vi "xiCam - GetParam_String.vi"(7 "PRM":T1, 8 "error in (no error)":errorcluster, 11 "xiCam In":refnum<k24>) -> (0 "error out":errorcluster, 3 "xiCam Out":refnum<k24>, 4 "String_Value":string)   [LabVIEW 2016]
doc: "This function returns parameters information (current value, minimum, maximum, info).\n\n<b>String GetParamString(string prm)</b>\nstring prm : Parameter name string. Use class PRM to set parameters.\nReturn : String value to be returned."
uses:
  C:/Users/Ries Lab/Documents/Microscope Control from Sheng Account/Microscope-Control/Device Library/Cameras/Ximea/xiLIB_64bit/xiLIB/xiCamLib/API/x64/xiApi.NETX64.dll
  API/x64/xiApi.NETX64.dll
  PRM/PRM/PRM_v2.ctl
  PRM/BUFF_POLICY/BUFF_POLICY.ctl
  PRM/DOWNSAMPLING_TYPE/DOWNSAMPLING_TYPE.ctl
  PRM/GPI_MODE/GPI_MODE.ctl
  PRM/GPO_MODE/GPO_MODE.ctl
  PRM/IMG_FORMAT/IMG_DATA_FORMAT.ctl
  PRM/LED_MODE/LED_MODE.ctl
  PRM/TRG_SOURCE/TRG_SOURCE.ctl
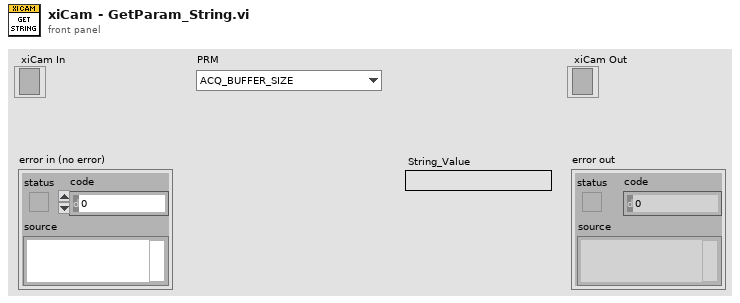
[diagram p1: front panel]
types:
  T1 = typedef "PRM_v2.ctl" = enum16{"ACQ_BUFFER_SIZE", "ACQ_FRAME_BURST_COUNT", "ACQ_TIMING_MODE", "ACQ_TRANSPORT_BUFFER_SIZE", "AE_MAX_LIMIT", "AEAG", "AEAG_LEVEL", "API_VERSION", "AG_MAX_LIMIT", "APPLY_CMS", "AUTO_BANDWIDTH_CALCULATION", "AUTO_WB", "AVAILABLE_BANDWIDTH", "AVAILABLE_BANDWIDTH_MAX", "AVAILABLE_BANDWIDTH_MIN", "BUFFER_POLICY", "BUFFERS_QUEUE_SIZE", "CC_MATRIX_00", "CC_MATRIX_01", "CC_MATRIX_02", "CC_MATRIX_03", "CC_MATRIX_10", "CC_MATRIX_11", "CC_MATRIX_12", "CC_MATRIX_13", "CC_MATRIX_20", "CC_MATRIX_21", "CC_MATRIX_22", "CC_MATRIX_23", "CC_MATRIX_30", "CC_MATRIX_31", "CC_MATRIX_32", "CC_MATRIX_33", "CHIP_TEMP", "CMS", "COLOR_FILTER_ARRAY", "COOLING", "DEBOUNCE_EN", "DEBOUNCE_POL", "DEBOUNCE_T0", "DEBOUNCE_T1", "DEBUG_LEVEL", "DEFAULT_CC_MATRIX", "DEVICE_INSTANCE_PATH", "DEVICE_MODEL_ID", "DEVICE_NAME", "DEVICE_SN", "DEVICE_TYPE", "DEVICE_USER_ID", "DOWNSAMPLING", "DOWNSAMPLING_TYPE", "DRV_VERSION", "EXP_PRIORITY", "EXPOSURE", "EXPOSURE_MAX", "EXPOSURE_MIN", "FFS_FILE_NAME", "FPGA1_VERSION", "FRAMERATE", "FRAMERATE_MAX", "FRAMERATE_MIN", "FREE_FFS_SIZE", "GAIN", "GAIN_MAX", "GAIN_MIN", "GAMMAC", "GAMMAY", "GPI_LEVEL", "GPI_MODE", "GPI_SELECTOR", "GPO_MODE", "GPO_SELECTOR", "HDR", "HDR_T1", "HDR_T2", "HEIGHT", "HEIGHT_MAX", "HEIGHT_MIN", "HOUSE_TEMP", "IMAGE_DATA_FORMAT", "IMAGE_IS_COLOR", "INPUT_CMS_PROFILE", "IS_COOLED", "IS_DEVICE_EXIST", "KNEEPOINT1", "KNEEPOINT2", "LED_MODE", "LED_SELECTOR", "LIMIT_BANDWIDTH", "LIMIT_BANDWIDTH_MAX", "LIMIT_BANDWIDTH_MIN", "LUT_EN", "LUT_INDEX", "LUT_INDEX_MAX", "LUT_INDEX_MIN", "LUT_VALUE", "LUT_VALUE_MAX", "LUT_VALUE_MIN", "MANUAL_WB", "MCU1_VERSION", "MCU2_VERSION", "OFFSET_X", "OFFSET_X_MAX", "OFFSET_X_MIN", "OFFSET_Y", "OFFSET_Y_MAX", "OFFSET_Y_MIN", "OUTPUT_CMS_PROFILE", "OUTPUT_DATA_BIT_DEPTH", "OUTPUT_DATA_PACKING", "READ_FILE_FFS", "RECENT_FRAME", "SENSOR_DATA_BIT_DEPTH", "SENSOR_MODE", "SENSOR_TAPS", "SHARPNESS", "SHUTTER_TYPE", "TARGET_TEMP", "TRG_DELAY", "TRG_SELECTOR", "TRG_SOFTWARE", "TRG_SOURCE", "USED_FFS_SIZE", "WB_KB", "WB_KG", "WB_KR", "WIDTH", "WIDTH_MAX", "WIDTH_MIN", "WRITE_FILE_FFS", "ACQ_BUFFER_SIZE_UNIT", "ACQ_TRANSPORT_BUFFER_COMMIT", "AEAG_ROI_HEIGHT", "AEAG_ROI_OFFSET_X", "AEAG_ROU_OFFSET_Y", "AEAG_ROI_WIDTH", "API_CONTEXT_LIST", "BINNING_HORIZONTAL", "BINNING_SELECTOR", "BINNING_VERTICAL", "COLUMN_FPN_CORRECTION", "COUNTER_SELECTOR", "COUNTER_VALUE", "DECIMATION_HORIZONTAL", "DECIMATION_SELECTOR", "DECIMATION_VERTICAL", "DEVICE_ID", "DEVICE_LOCATION_PATH", "DEVICE_MANIFEST", "DEVICE_RESET", "DEVICE_SENS_SN", "EXPOSURE_BURST_COUNT", "FFS_ACCESS_KEY", "GAIN_SELECTOR", "HW_REVISION", "IMAGE_BLACK_LEVEL", "IMAGE_DATA_BIT_DEPTH", "IMAGE_DATA_FORMAT_RGB32_ALPHA", "IMAGE_PAYLOAD_SIZE", "LENS_APERTURE_VALUE", "LENS_FEATURE", "LENS_FEATURE_SELECTOR", "LENS_FOCAL_LENGTH", "LENS_FOCUS_DISTANCE", "LENS_FOCUS_MOVE", "LENS_FOCUS_MOVEMENT_VALUE", "LENS_MODE", "OUTPUT_DATA_PACKING_TYPE", "SENSOR_CLOCK_FREQ_HZ", "SENSOR_CLOCK_FREQ_INDEX", "SENSOR_FEATURE_SELECTOR", "SENSOR_FEATURE_VALUE", "SENSOR_OUTPUT_CHANNEL_COUNT", "TRANSPORT_PIXEL_FORMAT", "TS_RST_MODE", "TS_RST_SOURCE", "SENS_DEFECTS_CORR_LIST_SELECTOR", "SENS_DEFECTS_CORR", "SENS_DEFECTS_CORR_LIST_CONTENT", "DEVICE_UNIT_SELECTOR", "DEVICE_UNIT_REGISTER_SELECTOR", "DEVICE_UNIT_REGISTER_VALUE"}
  T2 = typedef "BUFF_POLICY.ctl" = enum16{"UNSAFE", "SAFE"}
  T3 = typedef "DOWNSAMPLING_TYPE.ctl" = enum16{"BINNING", "SKIPPING"}
  T4 = typedef "GPI_MODE.ctl" = enum16{"OFF", "TRIGGER", "EXT_EVENT"}
  T5 = typedef "GPO_MODE.ctl" = enum16{"OFF", "ON", "FRAME_ACTIVE", "FRAME_ACTIVE_NEG", "EXPOSURE_ACTIVE", "EXPOSURE_ACTIVE_NEG"}
  T6 = typedef "IMG_DATA_FORMAT.ctl" = enum16{"MONO8", "MONO16", "RGB24", "RGB32", "RGBPLANAR", "RAW8", "RAW16"}
  T7 = typedef "LED_MODE.ctl" = enum16{"HEARTBEAT", "TRIGGER_ACTIVE", "EXT_EVENT_ACTIVE", "ACQUSITION", "EXPOSURE_ACTIVE", "FRAME_ACTIVE", "LINK", "OFF", "ON"}
  T8 = typedef "TRG_SOURCE.ctl" = enum16{"OFF", "EDGE_RISING", "EDGE_FALLING", "SOFTWARE"}
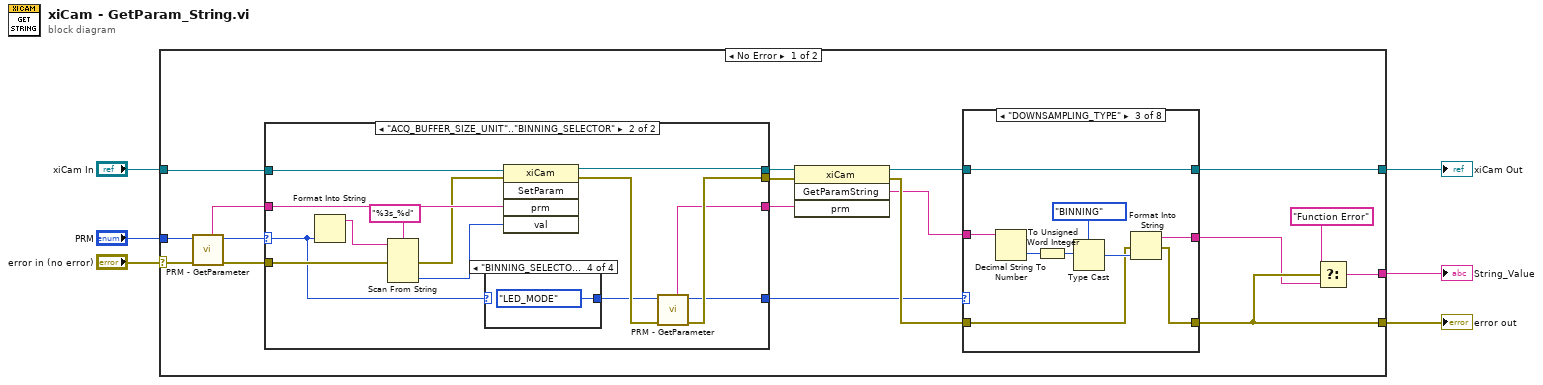
[diagram p0: block diagram]
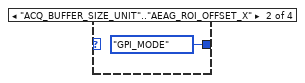
[diagram p4: hidden frame]
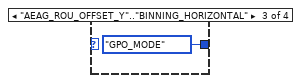
[diagram p5: hidden frame]
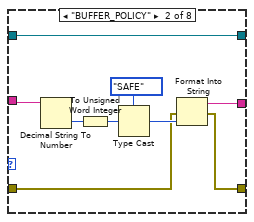
[diagram p7: hidden frame]
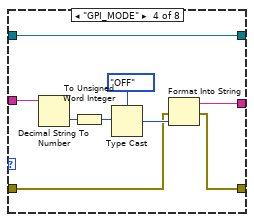
[diagram p8: hidden frame]
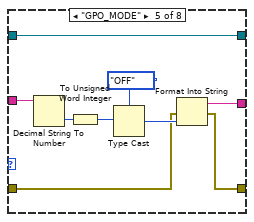
[diagram p9: hidden frame]
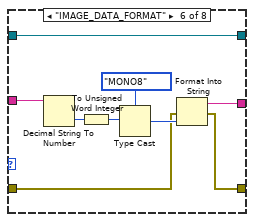
[diagram p10: hidden frame]
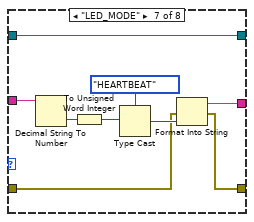
[diagram p11: hidden frame]
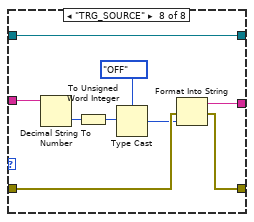
[diagram p12: hidden frame]
diagram:
  n1 = case shown="No Error" "error in (no error)" {
    selector: "error in (no error)" -> [w15 w112]
    tunnel: "xiCam In" -> [w17 w113]
    tunnel: [w21 w113] -> w4
    tunnel: [w10 w112] -> w3
    tunnel: "PRM" -> [w16 _]
    tunnel: [w8 _] -> w1
    frame No Error {
      n2 = call "PRM - GetParameter.vi"("error in (no error)"=w15, "PRM"=w16) -> ("error out"=w19:errorcluster, "PRM OUT"=w18:T1, "ParameterString"=w20:string)  [unwired: 7 in]
      n3 = case shown="\"ACQ_BUFFER_SIZE_UNIT\"..\"BINNING_SELECTOR\"" w18 {
        selector: w18 -> [w25 w34]
        tunnel: w20 -> [w26 w42]
        tunnel: w17 -> [w28 w41]
        tunnel: w19 -> [w27 w38]
        tunnel: [w28 w40] -> w14
        tunnel: [w27 w31] -> w13
        tunnel: [w26 w30] -> w12
        tunnel: [w25 w29] -> w11
        frame Default {
        }
        frame "ACQ_BUFFER_SIZE_UNIT".."BINNING_SELECTOR" {
          n4 = Format Into String(w34) -> (resulting string=w37:string)  [unwired: 3 in, 1 out]
          n5 = Scan From String(format string="%3s_%d", input string=w37, error in=w38) -> (error out=w35:errorcluster, output 2=w36:i32)  [unwired: 4 in, 2 out]
          n6 = case shown="\"BINNING_SELECTOR\"..\"DEVICE_RESET\"" w34 {
            tunnel: [_ PRM_v2."GPI_MODE" ("PRM") PRM_v2."GPO_MODE" ("PRM") PRM_v2."LED_MODE" ("PRM")] -> w32
            frame Default {
            }
            frame "ACQ_BUFFER_SIZE_UNIT".."AEAG_ROI_OFFSET_X" {
            }
            frame "AEAG_ROU_OFFSET_Y".."BINNING_HORIZONTAL" {
            }
            frame "BINNING_SELECTOR".."DEVICE_RESET" {
            }
          }
          n7 = invoke class="xiCam" method="SetParam"(reference=w41, error in=w35, "prm"=w42, "val"=w36) -> (reference out=w40:refnum<k24>, error out=w33:errorcluster)  [unwired: 1 in, 3 out]
          n8 = call "PRM - GetParameter.vi"("error in (no error)"=w33, "PRM"=w32) -> ("error out"=w31:errorcluster, "PRM OUT"=w29:T1, "ParameterString"=w30:string)  [unwired: 7 in]
        }
      }
      n9 = invoke class="xiCam" method="GetParamString"(reference=w14, error in=w13, "prm"=w12) -> (reference out=w23:refnum<k24>, error out=w24:errorcluster, "GetParamString"=w22:string)  [unwired: 1 in, 1 out]
      n10 = case shown="\"DOWNSAMPLING_TYPE\"" w11 {
        tunnel: w24 -> [w47 w54 w64 w73 w82 w91 w100 w110]
        tunnel: w23 -> [w48 w56 w66 w75 w84 w93 w102 w111]
        tunnel: w22 -> [w46 w51 w60 w69 w78 w87 w96 w107]
        tunnel: [w48 w56 w66 w75 w84 w93 w102 w111] -> w21
        tunnel: [w47 w53 w63 w72 w81 w90 w99 w109] -> w10
        tunnel: [w46 w52 w62 w71 w80 w89 w98 w108] -> w9
        frame Default {
        }
        frame "BUFFER_POLICY" {
          n11 = Decimal String To Number(string=w51) -> (number=w50:i32)  [unwired: 2 in, 1 out]
          n12 = To Unsigned Word Integer(number=w50) -> (unsigned 16bit integer=w49:u16)
          n13 = Type Cast(type=BUFF_POLICY."SAFE" ("BUFF_POLICY"), x=w49) -> (*(type *) &x=w55:T2)
          n14 = Format Into String(error in=w54, w55) -> (resulting string=w52:string, error out=w53:errorcluster)  [unwired: 2 in]
        }
        frame "DOWNSAMPLING_TYPE" {
          n15 = Decimal String To Number(string=w60) -> (number=w59:i32)  [unwired: 2 in, 1 out]
          n16 = To Unsigned Word Integer(number=w59) -> (unsigned 16bit integer=w58:u16)
          n17 = Type Cast(type=DOWNSAMPLING_TYPE."BINNING" ("Downsampling Type"), x=w58) -> (*(type *) &x=w65:T3)
          n18 = Format Into String(error in=w64, w65) -> (resulting string=w62:string, error out=w63:errorcluster)  [unwired: 2 in]
        }
        frame "GPI_MODE" {
          n19 = Decimal String To Number(string=w69) -> (number=w68:i32)  [unwired: 2 in, 1 out]
          n20 = To Unsigned Word Integer(number=w68) -> (unsigned 16bit integer=w67:u16)
          n21 = Type Cast(type=GPI_MODE."OFF" ("GPI_MODE"), x=w67) -> (*(type *) &x=w74:T4)
          n22 = Format Into String(error in=w73, w74) -> (resulting string=w71:string, error out=w72:errorcluster)  [unwired: 2 in]
        }
        frame "GPO_MODE" {
          n23 = Decimal String To Number(string=w78) -> (number=w77:i32)  [unwired: 2 in, 1 out]
          n24 = To Unsigned Word Integer(number=w77) -> (unsigned 16bit integer=w76:u16)
          n25 = Type Cast(type=GPO_MODE."OFF" ("GPO_MODE"), x=w76) -> (*(type *) &x=w83:T5)
          n26 = Format Into String(error in=w82, w83) -> (resulting string=w80:string, error out=w81:errorcluster)  [unwired: 2 in]
        }
        frame "IMAGE_DATA_FORMAT" {
          n27 = Decimal String To Number(string=w87) -> (number=w86:i32)  [unwired: 2 in, 1 out]
          n28 = To Unsigned Word Integer(number=w86) -> (unsigned 16bit integer=w85:u16)
          n29 = Type Cast(type=IMG_DATA_FORMAT."MONO8" ("IMG_FORMAT"), x=w85) -> (*(type *) &x=w92:T6)
          n30 = Format Into String(error in=w91, w92) -> (resulting string=w89:string, error out=w90:errorcluster)  [unwired: 2 in]
        }
        frame "LED_MODE" {
          n31 = Decimal String To Number(string=w96) -> (number=w95:i32)  [unwired: 2 in, 1 out]
          n32 = To Unsigned Word Integer(number=w95) -> (unsigned 16bit integer=w94:u16)
          n33 = Type Cast(type=LED_MODE."HEARTBEAT" ("LED_MODE"), x=w94) -> (*(type *) &x=w101:T7)
          n34 = Format Into String(error in=w100, w101) -> (resulting string=w98:string, error out=w99:errorcluster)  [unwired: 2 in]
        }
        frame "TRG_SOURCE" {
          n35 = Decimal String To Number(string=w107) -> (number=w106:i32)  [unwired: 2 in, 1 out]
          n36 = To Unsigned Word Integer(number=w106) -> (unsigned 16bit integer=w103:u16)
          n37 = Type Cast(type=TRG_SOURCE."OFF" ("TRG_SOURCE"), x=w103) -> (*(type *) &x=w104:T8)
          n38 = Format Into String(error in=w110, w104) -> (resulting string=w108:string, error out=w109:errorcluster)  [unwired: 2 in]
        }
      }
      n39 = Select(t="Function Error", s=w10, f=w9) -> (s? t:f=w8:string)
    }
    frame Error {
    }
  }
  "error out" <- w3
  "xiCam Out" <- w4
  "String_Value" <- w1
